vi "Init.vi"(8 "error in (no error)":errorcluster, 11 "Recipe View in":refnum<class "Recipe View.lvclass">) -> (0 "error out":errorcluster, 3 "Recipe View out":refnum<class "Recipe View.lvclass">)   [LabVIEW 2022 SP3, in "Recipe View.lvclass"]
uses:
  Recipe View.lvclass
  Data.ctl
  Recipe API/Recipe API.lvclass
  iView/base view/base view.lvclass
  Recipe View.lvclass/Recipe View.ctl
  Laser/Get Laser Status/Get Laser Status.lvclass
  IO Monitor/Get Daq Status/Get Daq Status.lvclass
  Camera/Camera Async Coms/Camera Async Coms.lvclass
  XY Stage/Interfaces/Async Coms/Async Coms.lvclass
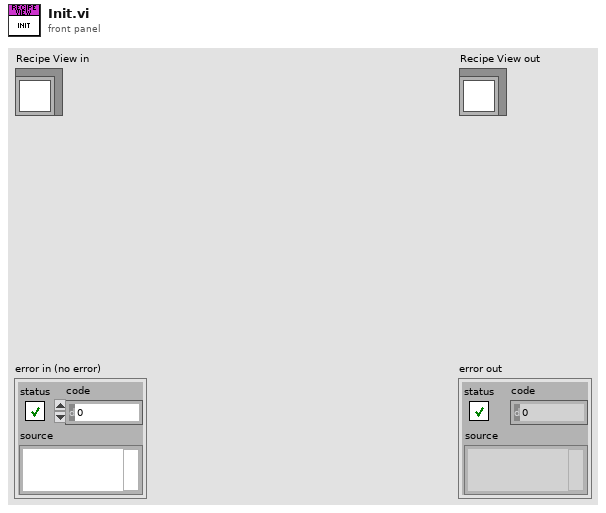
[diagram p1: front panel]
types:
  T1 = typedef "Recipe View.lvclass/Data.ctl" = cluster{"Recipe API.lvclass":refnum<class "Recipe API.lvclass">, "XY stage VIEW":refnum<class "base view.lvclass">, "Laser VIEW":refnum<class "base view.lvclass">, "Camera VIEW":refnum<class "base view.lvclass">, "DAQ VIEW":refnum<class "base view.lvclass">, "Stop":refnum<user-event>, "Camera Async Coms.lvclass":refnum<class "Camera Async Coms.lvclass">, "Get Daq Status.lvclass":refnum<class "Get Daq Status.lvclass">, "Get Laser Status.lvclass":refnum<class "Get Laser Status.lvclass">, "XY Stage Events.lvclass":refnum<class "Async Coms.lvclass">}
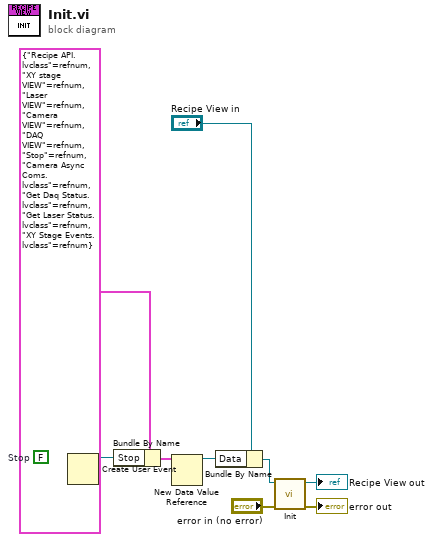
[diagram p0: block diagram]
diagram:
  w3 = FALSE  # Stop
  n1 = Create User Event(user event datatype=w3) -> (user event=w1:refnum<user-event>)  [unwired: 1 in, 1 out]
  n2 = Bundle By Name(cluster=T1 {"Recipe API.lvclass"=refnum, "XY stage VIEW"=refnum, "Laser VIEW"=refnum, "Camera VIEW"=refnum, "DAQ VIEW"=refnum, "Stop"=refnum, "Camera Async Coms.lvclass"=refnum, "Get Daq Status.lvclass"=refnum, "Get Laser Status.lvclass"=refnum, "XY Stage Events.lvclass"=refnum} ("Data"), "Stop"=w1) -> (w2:T1)
  n3 = New Data Value Reference(data value=w2) -> (data value reference=w4:refnum<data-value>)  [unwired: 1 in, 1 out]
  n4 = Bundle By Name(cluster="Recipe View in", "Data"=w4) -> (w5:refnum<class "Recipe View.lvclass">)
  n5 = call-parent "Init.vi"("error in (no error)"="error in (no error)", "base view in"=w5) -> ("error out"=→"error out":errorcluster, "base view out"=→"Recipe View out":refnum<class "Recipe View.lvclass">)  [unwired: 8 in]
